vi "Read Objects From Folder.vi"(8 "error in":errorcluster, 10 "Key":string, 11 "Archivist in":refnum<class "Archivist.lvclass">) -> (0 "error out":errorcluster, 1 "GUIDs":string[](array[string]), 2 "Object Settings Array":refnum<class "ObjectSettings.lvclass">[](array[class]), 3 "Archivist out":refnum<class "Archivist.lvclass">)   [LabVIEW 2019, in "Archivist.lvclass"]
uses:
  Archivist.lvclass
  Settings/ObjectSettings/ObjectSettings.lvclass
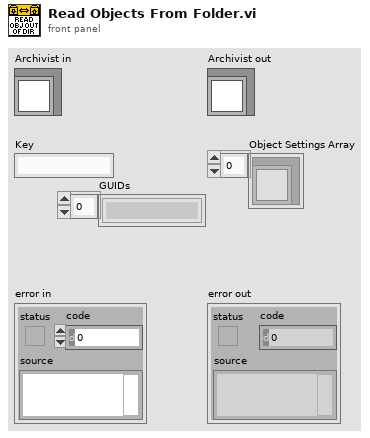
[diagram p1: front panel]
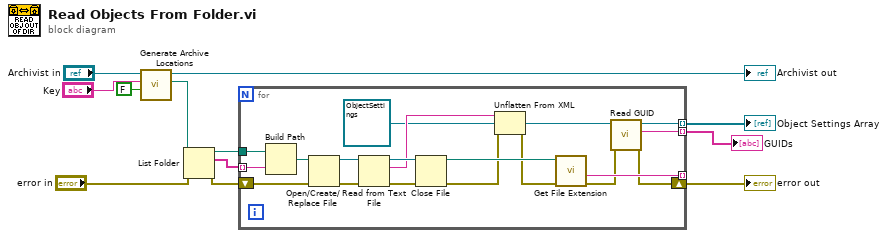
[diagram p0: block diagram]
diagram:
  n1 = call "Generate Archive Locations.vi"("Archive?"=FALSE, "Key"="Key", "Archivist In"="Archivist in") -> ("Path Out"=w8:path, "Archivist Out"=→"Archivist out":refnum<class "Archivist.lvclass">)  [unwired: 7 in]
  n2 = List Folder(path=w8, error in="error in") -> (path out=w7:path, filenames=w1:string[], error out=w6:errorcluster)  [unwired: 2 in, 1 out]
  n3 = for {
    tunnel: w1 -> [w30] mode=indexing
    tunnel: w7 -> [w31]
    tunnel: [w29] -> _ mode=indexing
    tunnel: [w20] -> w4 mode=indexing
    shift-right: [w19] -> w2
    shift-left: w6 -> [w14]
    tunnel: [w18] -> w5 mode=indexing
    n4 = Build Path(base path=w31, name or relative path=w30) -> (appended path=w28:path)
    n5 = Open/Create/Replace File(file path (use dialog)=w28, error in=w14) -> (refnum out=w27:refnum<file>, error out=w25:errorcluster)  [unwired: 4 in, 1 out]
    n6 = Read from Text File(file (use dialog)=w27, error in=w25) -> (refnum out=w26:refnum<file>, text=w23:string, error out=w24:errorcluster)  [unwired: 2 in, 1 out]
    n7 = Close File(refnum=w26, error in=w24) -> (path=w17:path, error out=w13:errorcluster)
    n8 = Unflatten From XML(xml string=w23, type=refnum<class "ObjectSettings.lvclass"> refnum ("ObjectSettings.lvclass"), error in (no error)=w13) -> (value=w21:refnum<class "ObjectSettings.lvclass">, error out=w16:errorcluster)
    n9 = call <vilib>:"Get File Extension.vi"("error in (no error)"=w16, "file"=w17) -> ("error out"=w15:errorcluster, "filename without extension"=w29:string)  [unwired: 5 in, 3 out]
    n10 = call-dynamic "Read GUID.vi"("error in (no error)"=w15, "ObjectSettings in"=w21) -> ("error out"=w19:errorcluster, "GUID"=w18:string, "ObjectSettings out"=w20:refnum<class "ObjectSettings.lvclass">)  [unwired: 7 in]
  }
  "error out" <- w2
  "Object Settings Array" <- w4
  "GUIDs" <- w5
